vi "Set Test Class.vi"(8 "error in (no error)":errorcluster, 10 "Class Name":string, 11 "Test in":refnum<class "Test.lvclass">) -> (0 "error out":errorcluster, 3 "Test out":refnum<class "Test.lvclass">)   [LabVIEW 2018, in "Test.lvclass"]
uses:
  Test.lvclass
  Test.lvclass/Test.ctl
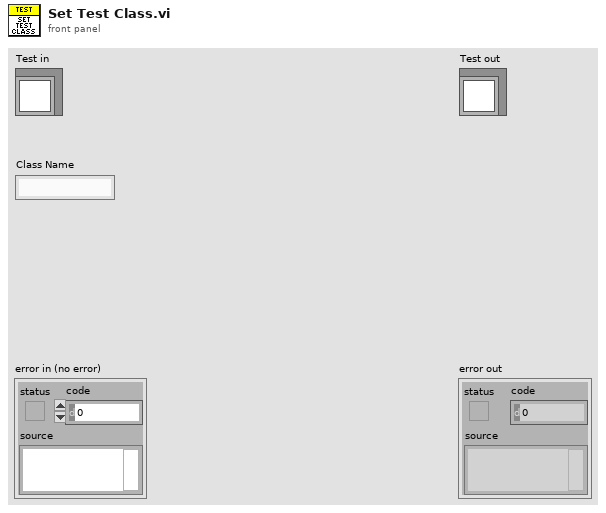
[diagram p1: front panel]
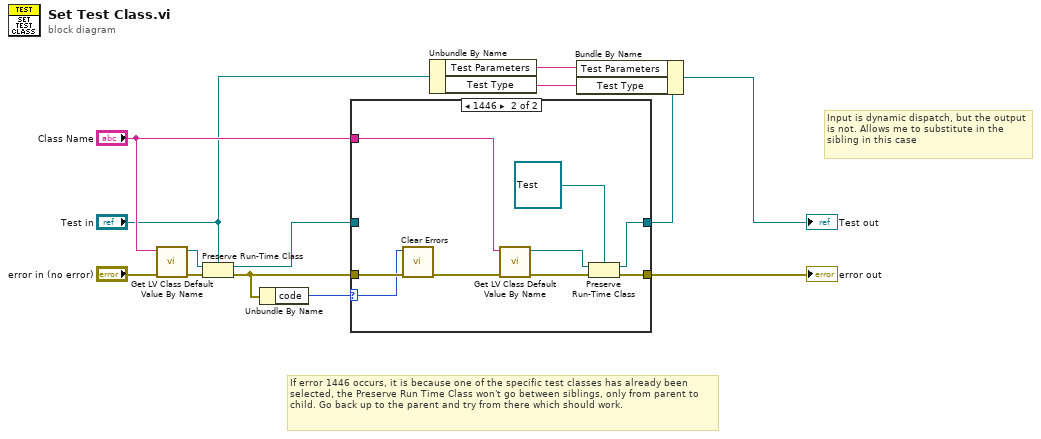
[diagram p0: block diagram]
diagram:
  # "Input is dynamic dispatch, but the output is not. Allows me to substitute in the sibling in this case"
  # "If error 1446 occurs, it is because one of the specific test classes has already been selected, the Preserve Run Time Class won't go between siblings, only from parent to child. Go back up to the parent and try from there which should work."
  n1 = call <vilib>:"Get LV Class Default Value By Name.vi"("error in (no error)"="error in (no error)", "class name"="Class Name") -> ("error out"=w12:errorcluster, "object"=w11:refnum<class>)  [unwired: 8 in]
  n2 = Preserve Run-Time Class(object in=w11, error in=w12, 2:"Test in") -> (object out=w9:refnum<class "Test.lvclass">, error out=w6:errorcluster)
  n3 = Unbundle By Name(w6) -> ("code"=w10:i32)
  n4 = case shown="1446" w10 {
    selector: w10 -> [_ w17]
    tunnel: w9 -> [w15 _]
    tunnel: [w15 w19] -> w8
    tunnel: [w14 w18] -> w7
    tunnel: w6 -> [w14 w23]
    tunnel: "Class Name" -> [_ w21]
    frame Default {
    }
    frame 1446 {
      n5 = call <vilib>:"Clear Errors.vi"("error in (no error)"=w23, "specific error code to clear (0: all)"=w17) -> ("error out"=w22:errorcluster)  [unwired: 4 in, 1 out]
      n6 = call <vilib>:"Get LV Class Default Value By Name.vi"("error in (no error)"=w22, "class name"=w21) -> ("error out"=w24:errorcluster, "object"=w20:refnum<class>)  [unwired: 8 in]
      n7 = Preserve Run-Time Class(object in=w20, error in=w24, 2:refnum<class "Test.lvclass"> refnum ("Test.lvclass")) -> (object out=w19:refnum<class "Test.lvclass">, error out=w18:errorcluster)
    }
  }
  "error out" <- w7
  n8 = Unbundle By Name("Test in") -> ("Test Parameters"=w2:string, "Test Type"=w1:string)
  n9 = Bundle By Name(cluster=w8, "Test Parameters"=w2, "Test Type"=w1) -> (→"Test out":refnum<class "Test.lvclass">)
